vi "Thb per direction.vi"(1 "Done?":cluster{"x":bool, "y":bool, "th":bool}, 2 "Direction":T2(ring), 3 "Tbh data":T1, 4 "Invert value":cluster{"x":bool, "y":bool, "th":bool}) -> (0 "Velocity Ajustment":dbl)   [LabVIEW 2023]
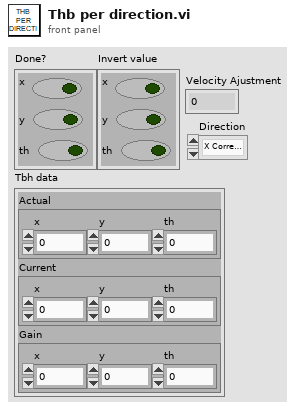
[diagram p1: front panel]
types:
  T1 = cluster{"Actual":cluster{"x":dbl, "y":dbl, "th":dbl}, "Current":cluster{"x":dbl, "y":dbl, "th":dbl}, "Gain":cluster{"x":dbl, "y":dbl, "th":dbl}}
  T2 = enum16{"X Correction", "Y Correction", "Theta Correction"}
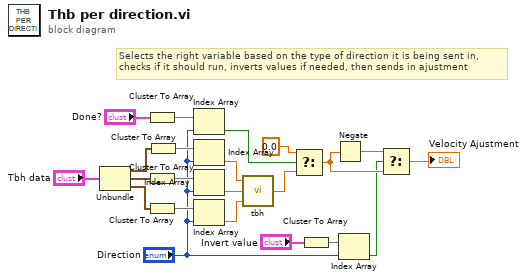
[diagram p0: block diagram]
diagram:
  # "Selects the right variable based on the type of direction it is being sent in, \nchecks if it should run, inverts values if needed, then sends in ajustment"
  n1 = Unbundle("Tbh data") -> ("Actual"=w3:cluster{"x":dbl, "y":dbl, "th":dbl}, "Current"=w2:cluster{"x":dbl, "y":dbl, "th":dbl}, "Gain"=w1:cluster{"x":dbl, "y":dbl, "th":dbl})
  n2 = Cluster To Array(cluster="Done?") -> (array=w8:bool[])
  n3 = Cluster To Array(cluster=w2) -> (array=w14:dbl[])
  n4 = Cluster To Array(cluster=w1) -> (array=w15:dbl[])
  n5 = Cluster To Array(cluster=w3) -> (array=w16:dbl[])
  n6 = Index Array(array=w8, index="Direction") -> (element=w7:bool)
  n7 = Index Array(array=w16, index="Direction") -> (element=w10:dbl)
  n8 = Index Array(array=w14, index="Direction") -> (element=w11:dbl)
  n9 = Index Array(array=w15, index="Direction") -> (element=w13:dbl)
  n10 = call "tbh.vi"("Gain"=w13, "Act"=w11, "Cmd"=w10) -> ("Out"=w19:dbl)
  n11 = Select(t=0.0, s=w7, f=w19) -> (s? t:f=w21:dbl)
  n12 = Cluster To Array(cluster="Invert value") -> (array=w17:bool[])
  n13 = Negate(x=w21) -> (-x=w22:dbl)
  n14 = Index Array(array=w17, index="Direction") -> (element=w12:bool)
  n15 = Select(t=w22, s=w12, f=w21) -> (s? t:f=→"Velocity Ajustment":dbl)
